vi "PH_Class.constructor.vi"(0 "name":string, 2 "data in":string, 5 "error in":errorcluster) -> (14 "i ref out":refnum<vi>, 16 "data out":string, 19 "error out":errorcluster)   [LabVIEW 2014, in "PH_Class.lvlib"]
doc: "This class is forseen to be inherited from. With its help data of devices can be stored in the PHELIX shot data base (PSDB). \n\n\n\nauthor: Stefan Götte, GSI\n\nLicense Agreement for this software:\n\nCopyright (C)\nGesellschaft für Schwerionenforschung, GSI\nPlanckstr. 1\n64291 Darmstadt\nGermany\n\nContact: D.Beck@gsi.de \n\nThis program is free software; you can redistribute it and/or modify it under the terms of the \nGNU General Public License as published by the Free Software Foundation; either version 2 of \nthe license, or (at your option) any later version.\n\nThis program is distributed in the hope that it will be useful, but WITHOUT ANY WARRANTY; \nwithout even the implied warranty of MERCHANTABILITY or FITNESS FOR A PARTICULAR PURPOSE. See the GNU General License for more details (http://www.gnu.org).\n\nGesellschaft für Schwerionenforschung, GSI\nPlanckstr. 1, 64291 Darmstadt, Germany\nFor all questions and ideas contact: M.Richter@gsi.de, H.Brand@gsi.de or D.Beck@gsi.de.\nLast update: 16-JUN-2004"
uses:
  PH_Class.lvlib
  PH_Class.i attribute.ctl
  CSCore/BaseGUI/BaseGUI.lvlib
  PH_Common/PH_Common.lvlib
  CSCore/CSSystem/CSSystemLib/CSSystemLib.lvlib
  CSCore/BaseProcess/BaseProcess.lvlib
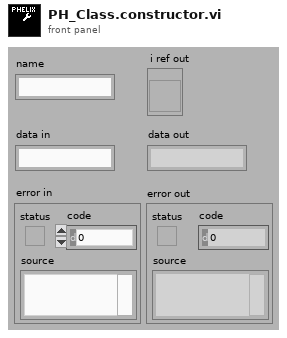
[diagram p1: front panel]
types:
  T1 = enum16{"SetAttribute", "GetAttribute", "CreateAttribute", "DestroyAttribute", "DestroyAllAtributes"}
  T2 = typedef "PH_Class.lvlib/PH_Class.i attribute.ctl" = cluster{"Event":refnum<user-event>, "Event registered":refnum<k4>, "GUI Refs stored":refnum<k4>}
  T3 = typedef "BaseProcess.lvlib/BaseProcess.i attribute.ctl" = cluster{"EventStatus":string, "EventError":i32, "PresetEvtWatchD":i32, "PresetPdcWatchD":i32, "EventTimeout":i32, "PeriodicInterval":i32, "Interface":string[], "Address":string[], "Special":string[], "PeriodicError":i32, "PeriodicStatus":string, "SuperProc":string, "Descriptors":T4[], "CaseRef":refnum<vi>, "PdcRef":refnum<vi>, "Thread Ref":refnum<vi>, "eventErrorID":i32, "eventStatusID":i32, "periodicErrorID":i32, "periodicStatusID":i32, "pdcCtrID":i32}
  T4 = typedef "BaseProcess.lvlib/BaseProcess.descriptor definition.ctl" = cluster{"selector":string, "descriptor":T5}
  T5 = typedef "BaseProcess.lvlib/BaseProcess.descriptor string definition.ctl" = string
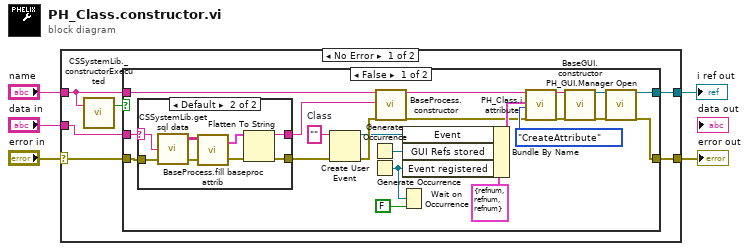
[diagram p0: block diagram]
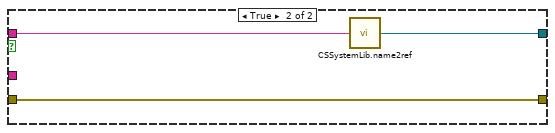
[diagram p3: hidden frame]
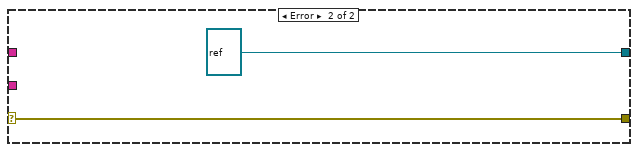
[diagram p4: hidden frame]
diagram:
  n1 = case shown="No Error" "error in" {
    selector: "error in" -> [w11 w47]
    tunnel: [w8 refnum<vi> refnum ("i ref out")] -> w5
    tunnel: [w9 w47] -> w4
    tunnel: "name" -> [w7 _]
    tunnel: "data in" -> [w10 _]
    frame No Error {
      n2 = call "CSSystemLib._constructorExecuted.vi"("name"=w7) -> ("constructor executed?"=w6:bool)  [unwired: 18 in]
      n3 = case shown="False" w6 {
        tunnel: w11 -> [w17 w43]
        tunnel: w10 -> [w12 _]
        tunnel: w7 -> [w24 w45]
        tunnel: [w30 w43] -> w9
        tunnel: [w31 w44] -> w8
        frame False {
          w23 = ""  # Class
          n4 = case shown="Default" w12 {
            selector: w12 -> [w33 w35]
            tunnel: w17 -> [w34 w40]
            tunnel: [w34 w38] -> w16
            tunnel: [w33 w36] -> w15
            frame "", "N/A" {
            }
            frame Default {
              n5 = call "CSSystemLib.get sql data.vi"("error in (no error)"=w40, "object"=w35) -> ("error out"=w42:errorcluster, "queryResults"=w41:string[][])  [unwired: 1 in, 1 out]
              n6 = call "BaseProcess.fill baseproc attrib.vi"("error in (no error)"=w42, "queryResults"=w41) -> ("error out"=w39:errorcluster, "cluster out"=w37:T3)  [unwired: 1 in]
              n7 = Flatten To String(anything=w37, error in (no error)=w39) -> (data string=w36:string, error out=w38:errorcluster)  [unwired: 2 in, 1 out]
            }
          }
          n8 = Create User Event(user event datatype=w23, error in=w16) -> (user event=w21:refnum<user-event>, error out=w22:errorcluster)
          n9 = Generate Occurrence() -> (w20:refnum<k4>)
          n10 = Generate Occurrence() -> (w19:refnum<k4>)
          n11 = call "BaseProcess.constructor.vi"("name"=w24, "data in"=w15, "error in (no error)"=w22) -> ("i ref out"=w13:refnum<vi>, "error out"=w14:errorcluster)  [unwired: 14 in, 1 out]
          n12 = Wait on Occurrence(1:FALSE ("ignore previous (T)"), 2:w19) -> ()  [unwired: 1 in, 1 out]
          n13 = Bundle By Name(cluster=T2 {"Event"=refnum, "Event registered"=refnum, "GUI Refs stored"=refnum} ("CLASS.i attribute"), "Event"=w21, "GUI Refs stored"=w20, "Event registered"=w19) -> (w28:T2)
          n14 = call "PH_Class.i attribute.vi"("VI Refnum"=w13, "CLASS.i attribute"=w28, "Action"=T1."CreateAttribute", "error in (no error)"=w14) -> ("error out"=w26:errorcluster)  [unwired: 13 in, 2 out]
          n15 = call "BaseGUI.constructor.vi"("name"=w24, "error in (no error)"=w26) -> ("i ref out"=w27:refnum<vi>, "error out"=w25:errorcluster)  [unwired: 15 in, 1 out]
          n16 = call "PH_GUI.Manager Open.vi"("i ref in"=w27, "error in"=w25) -> ("i ref out"=w31:refnum<vi>, "error out"=w30:errorcluster)  [unwired: 16 in]
        }
        frame True {
          n17 = call "CSSystemLib.name2ref.vi"("name"=w45) -> ("obj refnum"=w44:refnum<vi>)
        }
      }
    }
    frame Error {
    }
  }
  "i ref out" <- w5
  "error out" <- w4
